vi "Spectrum Measurement.vi"() -> ()   [LabVIEW 2013]
uses:
  <vilib>/Analysis/4window.llb/windowTd.ctl
  <vilib>/measure/maspectr.llb/FFT Spectrum (Mag-Phase) for 1 Chan.vi
  <vilib>/measure/NI_MABase.lvlib
  <vilib>/measure/NI_MAPro.lvlib
  <vilib>/Analysis/NI_AALPro.lvlib
panel:
  in  "window":T1=1 items=["Rectangle"=0, "Hanning"=1, "Hamming"=2, "Blackman-Harris"=3, "Exact Blackman"=4, "Blackman"=5, "Flat Top"=6, "4 Term B-Harris "=7, "7 Term B-Harris"=8, "Low Sidelobe"=9, "Blackman Nuttall"=11, "Triangle"=30, "Bartlett-Hanning"=31, "Bohman"=32, "Parzen"=33, "Welch"=34, "Kaiser"=60, "Dolph-Chebyshev"=61, "Gaussian"=62]
  in  "stop":bool
  out "Waveform Graph":cluster{"f0":dbl, "df":dbl, "magnitude":dbl[]}(graph)
  in  "Enum":T2(ring)
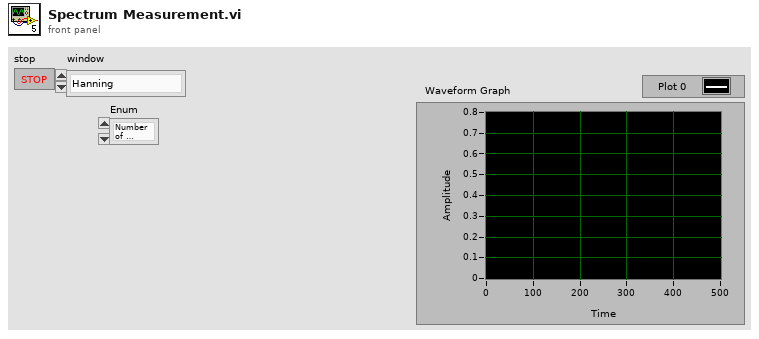
[diagram p1: front panel]
types:
  T1 = typedef "NI_AALPro.lvlib/windowTd.ctl" = u32
  T2 = enum16{"Number of Samples=100", "Number of Samples=1000"}
  T3 = cluster{"dB On (F)":bool, "unwrap phase (F)":bool, "convert to degree (F)":bool}
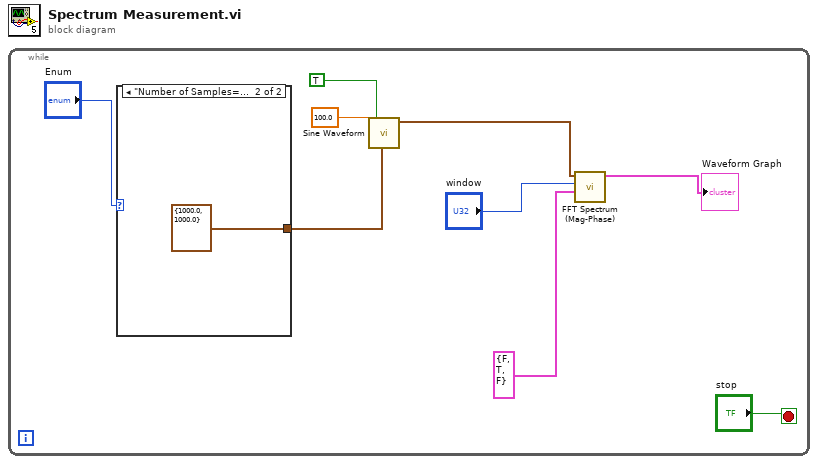
[diagram p0: block diagram]
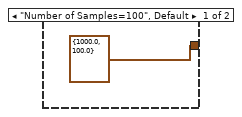
[diagram p2: hidden frame]
diagram:
  n1 = while {
    stop <- "stop" stop-if-true
    n2 = case shown="\"Number of Samples=1000\"" "Enum" {
      tunnel: [cluster{"Fs":dbl, "#s":dbl} {"Fs"=1000.0, "#s"=100.0} ("sampling info") cluster{"Fs":dbl, "#s":dbl} {"Fs"=1000.0, "#s"=1000.0} ("sampling info")] -> w5
      frame "Number of Samples=100", Default {
      }
      frame "Number of Samples=1000" {
      }
    }
    n3 = call <vilib>:"Sine Waveform.vi"("sampling info"=w5, "reset signal"=TRUE, "frequency"=100.0) -> ("signal out"=w4:waveform(dbl))  [unwired: 7 in, 1 out]
    n4 = call-poly <vilib>:"FFT Spectrum (Mag-Phase).vi"("view"=T3 {"dB On (F)"=FALSE, "unwrap phase (F)"=TRUE, "convert to degree (F)"=FALSE}, "window"="window", "time signal"=w4) -> ("magnitude"=→"Waveform Graph":cluster{"f0":dbl, "df":dbl, "magnitude":dbl[]})  [unwired: 4 in, 4 out]
  }
